vi "BLAS3 Utility.vi"   [LabVIEW 2018, in "NI_AALBLAS.lvlib"]
uses:
  NI_AALBLAS.lvlib
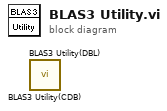
[diagram p0: block diagram]
diagram:
  n1 = call "BLAS3 Utility(CDB).vi"() -> ()  [unwired: 14 in, 6 out]
  n2 = call "BLAS3 Utility(DBL).vi"() -> ()  [unwired: 14 in, 6 out]
